vi "SS Class Init.vi"(7 "VI Refnum":refnum<vi>, 8 "error in (no error)":errorcluster, 9 "Init Data":variant, 10 "Device":string, 11 "Subsystem Pressure Monitor in":refnum<class "Subsystem Pressure Monitor.lvclass">) -> (0 "error out":errorcluster, 2 "Channel List":refnum<class "HK Item.lvclass">[](array[class]), 3 "Subsystem Pressure Monitor out":refnum<class "Subsystem Pressure Monitor.lvclass">)   [LabVIEW 2024, in "Subsystem Pressure Monitor.lvclass"]
uses:
  Subsystem Pressure Monitor.lvclass
  hk-channel-class/hk-channel-class/HK Item/HK Item.lvclass
  Subsystem Class.lvclass
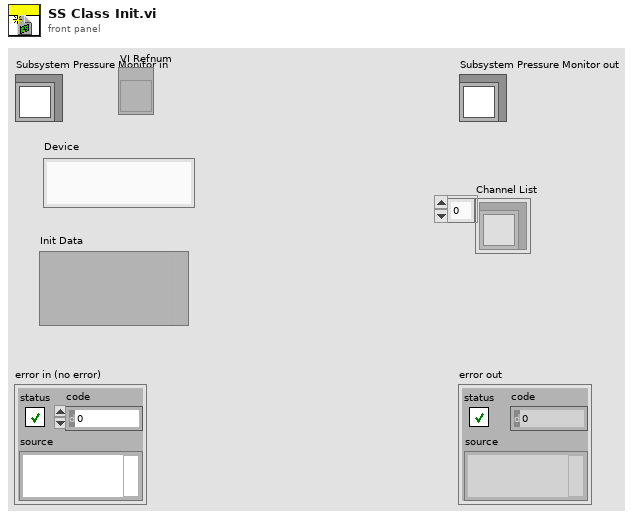
[diagram p1: front panel]
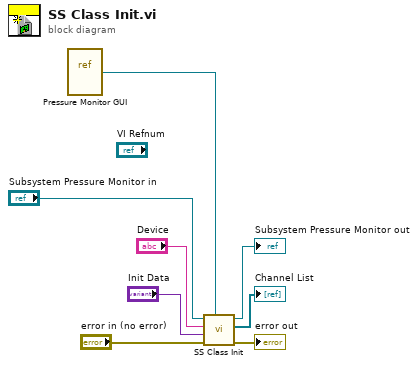
[diagram p0: block diagram]
diagram:
  n1 = vi-ref "Pressure Monitor GUI.vi"() -> (w1:refnum<vi>)
  n2 = call-parent "SS Class Init.vi"("VI Refnum"=w1, "error in (no error)"="error in (no error)", "Init Data"="Init Data", "Device"="Device", "Subsystem Class in"="Subsystem Pressure Monitor in") -> ("error out"=→"error out":errorcluster, "Channel List"=→"Channel List":refnum<class "HK Item.lvclass">[], "Subsystem Class out"=→"Subsystem Pressure Monitor out":refnum<class "Subsystem Pressure Monitor.lvclass">)  [unwired: 4 in]
